vi "TestPFGVRequests.vi"(10 "PUID":string="d1") -> (0 "error out":errorcluster, 2 "Pass":bool)   [LabVIEW 2015]
uses:
  TypeDef/PersonnelActions.ctl
  LVClasses/Request/PersonnelType.ctl
  LVClasses/Request/RequestType.ctl
  LVClasses/Request/Request.lvclass/Request.ctl
  LVClasses/Request/Read Summary.vi
  LVClasses/Request/Request.lvclass
panel:
  out "Remove":bool
  out "Add":bool
  out "Add Request 2":string
  out "Read Request 2":string
  out "Remove Request":string
  out "Add Request 1":string
  out "Read Requests 1":string
  out "Read Requests 2":string
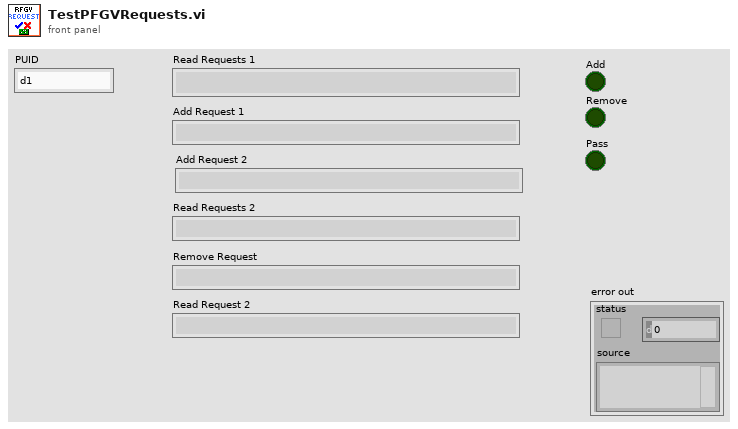
[diagram p1: front panel]
types:
  T1 = typedef "Request.lvclass/RequestType.ctl" = enum16{"Specific Call To Room", "General Call To Room"}
  T2 = typedef "Request.lvclass/PersonnelType.ctl" = u16
  T3 = typedef "PersonnelActions.ctl" = enum16{"Init", "Read Personnel", "Add Personnel", "Remove Personnel", "Read Name", "Write Name", "Read Role", "Write Role", "Read Requests", "Add Requests", "Remove Requests", "Read PUIDs", "Read PUIDs for Role", "Read All Personnel"}
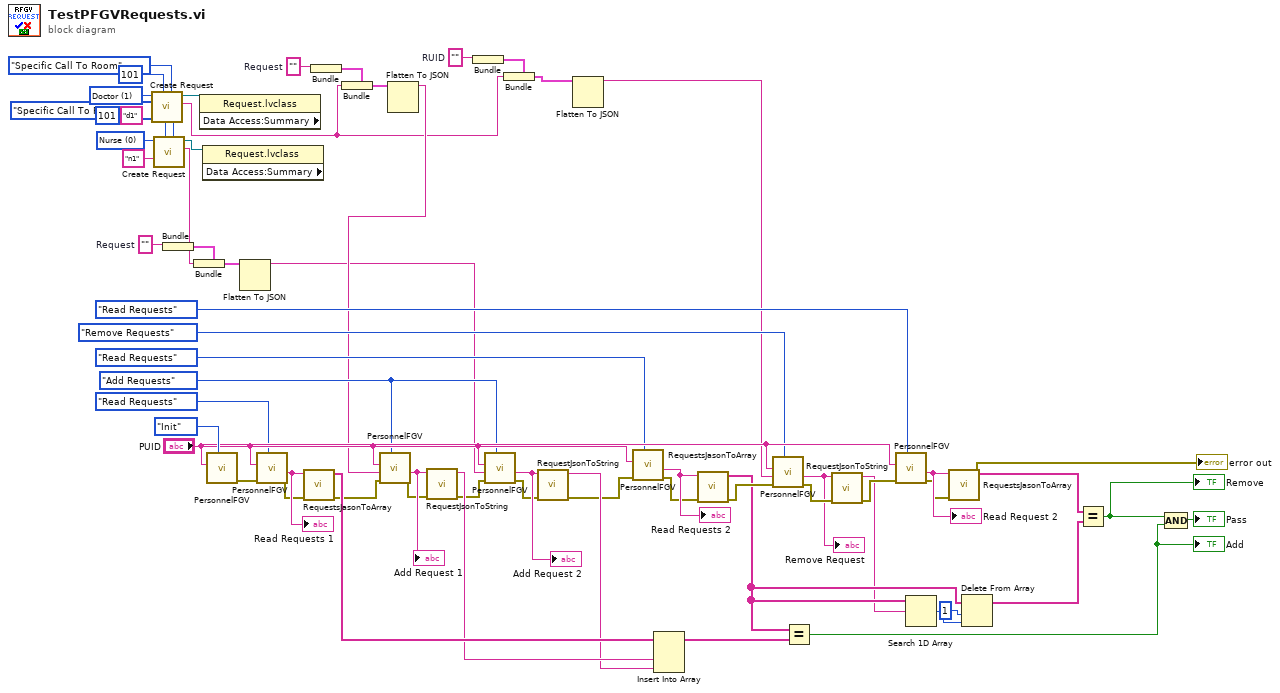
[diagram p0: block diagram]
diagram:
  w6 = ""  # RUID
  w15 = T2 0 items=["Nurse", "Doctor", "Cleanning", "Admin"] ("Personnel Type")
  w16 = T2 1 items=["Nurse", "Doctor", "Cleanning", "Admin"] ("Personnel Type")
  w48 = PersonnelActions."Add Requests" ("Actions")
  w55 = ""  # Request
  w62 = ""  # Request
  n1 = call "Create Request.vi"("Request Type"=RequestType."Specific Call To Room", "Room Number"=101, "Name"="d1", "Personnel Type"=w16) -> ("RUID"=w1:string, "Request out"=w17:refnum<class "Request.lvclass">)  [unwired: 5 in, 1 out]
  n2 = call "Create Request.vi"("Request Type"=RequestType."Specific Call To Room", "Room Number"=101, "Name"="n1", "Personnel Type"=w15) -> ("RUID"=w2:string, "Request out"=w18:refnum<class "Request.lvclass">)  [unwired: 5 in, 1 out]
  n3 = Bundle("Request"=w55) -> (w56:cluster{"Request":string})  [unwired: 1 in]
  n4 = Bundle(cluster=w56, "Request"=w2) -> (w57:cluster{"Request":string})
  n5 = property class="Request.lvclass" props=["Data Access:Summary"](reference=w17) -> ()  [unwired: 1 in, 3 out]
  n6 = property class="Request.lvclass" props=["Data Access:Summary"](reference=w18) -> ()  [unwired: 1 in, 3 out]
  n7 = call "PersonnelFGV.vi"("Actions"=PersonnelActions."Init", "PUID"="PUID") -> ("error out"=w63:errorcluster)  [unwired: 8 in, 1 out]
  n8 = Flatten To JSON(anything=w57) -> (JSON string=w7:string)  [unwired: 2 in, 1 out]
  n9 = call "PersonnelFGV.vi"("Actions"=PersonnelActions."Read Requests", "error in (no error)"=w63, "PUID"="PUID") -> ("error out"=w39:errorcluster, "Data Out"=w45:string)  [unwired: 7 in]
  "Read Requests 1" <- w45
  n10 = call "RequestsJasonToArray.vi"("error in (no error)"=w39, "Data Out"=w45) -> ("error out"=w38:errorcluster, "REQs"=w44:string[])  [unwired: 8 in]
  n11 = Bundle("Request"=w62) -> (w61:cluster{"Request":string})  [unwired: 1 in]
  n12 = Bundle(cluster=w61, "Request"=w1) -> (w60:cluster{"Request":string})
  n13 = Flatten To JSON(anything=w60) -> (JSON string=w8:string)  [unwired: 2 in, 1 out]
  n14 = call "PersonnelFGV.vi"("Actions"=w48, "error in (no error)"=w38, "Data In"=w8, "PUID"="PUID") -> ("error out"=w37:errorcluster, "Data Out"=w47:string)  [unwired: 6 in]
  "Add Request 1" <- w47
  n15 = call "RequestJsonToString.vi"("error in (no error)"=w37, "Data Out"=w47) -> ("error out"=w36:errorcluster, "Request"=w43:string)  [unwired: 8 in]
  n16 = Bundle("RUID"=w6) -> (w5:cluster{"RUID":string})  [unwired: 1 in]
  n17 = call "PersonnelFGV.vi"("Actions"=w48, "error in (no error)"=w36, "Data In"=w7, "PUID"="PUID") -> ("error out"=w35:errorcluster, "Data Out"=w46:string)  [unwired: 6 in]
  "Add Request 2" <- w46
  n18 = Bundle(cluster=w5, "RUID"=w1) -> (w4:cluster{"RUID":string})
  n19 = call "RequestJsonToString.vi"("error in (no error)"=w35, "Data Out"=w46) -> ("error out"=w34:errorcluster, "Request"=w42:string)  [unwired: 8 in]
  n20 = Flatten To JSON(anything=w4) -> (JSON string=w3:string)  [unwired: 2 in, 1 out]
  n21 = call "PersonnelFGV.vi"("Actions"=PersonnelActions."Read Requests", "error in (no error)"=w34, "PUID"="PUID") -> ("error out"=w33:errorcluster, "Data Out"=w41:string)  [unwired: 7 in]
  "Read Requests 2" <- w41
  n22 = Insert Into Array(array=w44, new element #1=w43, new element #2=w42) -> (w40:string[])  [unwired: 1 in]
  n23 = call "RequestsJasonToArray.vi"("error in (no error)"=w33, "Data Out"=w41) -> ("error out"=w32:errorcluster, "REQs"=w26:string[])  [unwired: 8 in]
  n24 = call "PersonnelFGV.vi"("Actions"=PersonnelActions."Remove Requests", "error in (no error)"=w32, "Data In"=w3, "PUID"="PUID") -> ("error out"=w31:errorcluster, "Data Out"=w29:string)  [unwired: 6 in]
  "Remove Request" <- w29
  n25 = Equal?(x=w26, y=w40) -> (x = y?=w58:bool)
  "Add" <- w58
  n26 = call "RequestJsonToString.vi"("error in (no error)"=w31, "Data Out"=w29) -> ("error out"=w30:errorcluster, "Request"=w25:string)  [unwired: 8 in]
  n27 = call "PersonnelFGV.vi"("Actions"=PersonnelActions."Read Requests", "error in (no error)"=w30, "PUID"="PUID") -> ("error out"=w23:errorcluster, "Data Out"=w24:string)  [unwired: 7 in]
  "Read Request 2" <- w24
  n28 = Search 1D Array(1D array=w26, element=w25) -> (index of element=w28:i32)  [unwired: 1 in]
  n29 = call "RequestsJasonToArray.vi"("error in (no error)"=w23, "Data Out"=w24) -> ("error out"=→"error out":errorcluster, "REQs"=w21:string[])  [unwired: 8 in]
  n30 = Delete From Array(array=w26, length=1, index=w28) -> (array with subset deleted=w20:string[])  [unwired: 1 out]
  n31 = Equal?(x=w21, y=w20) -> (x = y?=w59:bool)
  "Remove" <- w59
  n32 = Compound Arithmetic op=AND(w59, w58) -> (→"Pass":bool)
